vi "Clear.vi"(8 "error in (no error)":errorcluster, 11 "Low Level PSU In":refnum<class "Low Level PSU.lvclass">) -> (0 "error out":errorcluster, 3 "Low Level PSU Out":refnum<class "Low Level PSU.lvclass">)   [LabVIEW 2020, in "Low Level PSU.lvlib" / "Low Level PSU.lvclass"]
uses:
  Low Level PSU.lvclass
  Low Level PSU.lvclass/Low Level PSU.ctl
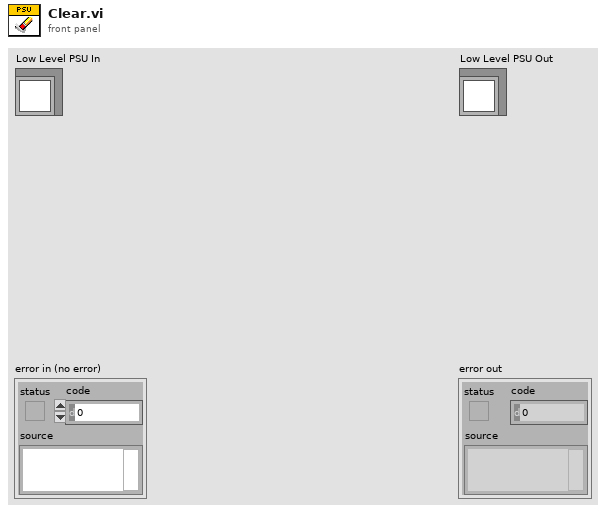
[diagram p1: front panel]
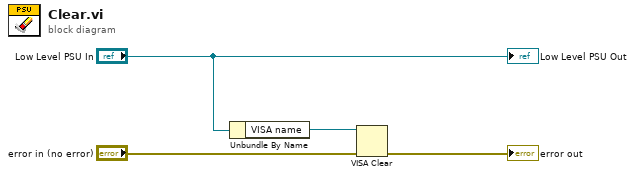
[diagram p0: block diagram]
diagram:
  n1 = Unbundle By Name("Low Level PSU In") -> ("VISA name"=w1:refnum<visa-resource-name>)
  n2 = VISA Clear(VISA resource name=w1, error in (no error)="error in (no error)") -> (error out=→"error out":errorcluster)  [unwired: 1 out]
  "Low Level PSU Out" <- "Low Level PSU In"
